vi "pointage.vi"() -> ()   [LabVIEW 2024]
uses:
  <vilib>/drjdpowell/SQLite Library/SQL Connection/Open (string).vi
  <vilib>/drjdpowell/SQLite Library/SQL Connection/Execute SQL (No results).vi
  <vilib>/drjdpowell/SQLite Library/SQL Connection/Execute SQL.vi
  <vilib>/drjdpowell/SQLite Library/SQL Connection/Connection.lvclass
  <vilib>/drjdpowell/SQLite Library/SQLite.lvlib
panel:
  out "Données pointage":string[][](table)
  out "Heure":string
  out "Identifiant":dbl
  in  "Heure":timestamp
  in  "Identifiant":dbl
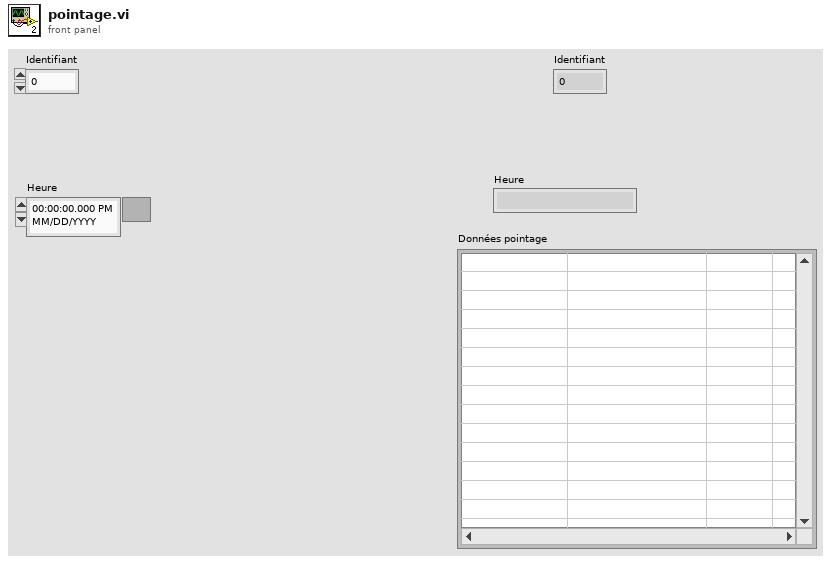
[diagram p1: front panel]
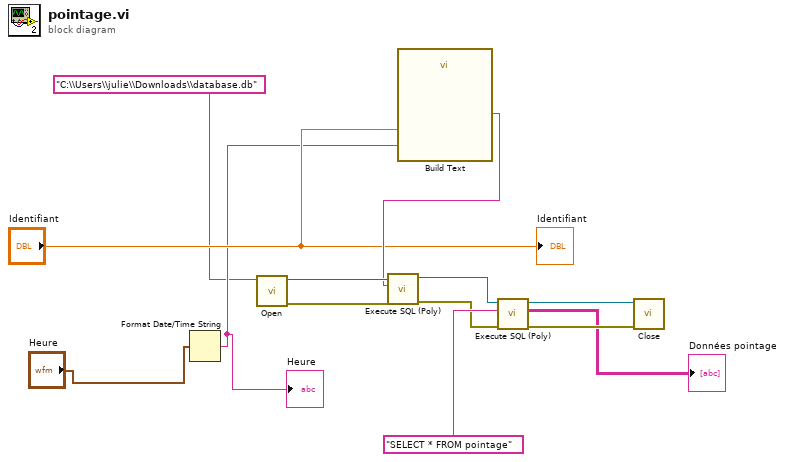
[diagram p0: block diagram]
diagram:
  n1 = Format Date/Time String(seconds (now)="Heure") -> (date/time string=w8:string)  [unwired: 2 in]
  "Heure" <- w8
  n2 = call-poly <vilib>:"Open.vi"("db file"="C:\\Users\\julie\\Downloads\\database.db") -> ("error out"=w11:errorcluster, "SQLite Connection"=w12:refnum<class "Connection.lvclass">)  [unwired: 9 in]
  n3 = call "Build Text"("id"="Identifiant", "heure"=w8) -> ("Result"=w10:string)  [unwired: 12 in, 1 out]
  n4 = call-poly <vilib>:"Execute SQL (Poly).vi"("error in (no error)"=w11, "SQL"=w10, "SQLite Connection in"=w12) -> ("error out"=w1:errorcluster, "SQLite Connection"=w2:refnum<class "Connection.lvclass">)  [unwired: 7 in]
  n5 = call-poly <vilib>:"Execute SQL (Poly).vi"("error in (no error)"=w1, "SQL"="SELECT * FROM pointage", "SQLite Connection in"=w2) -> ("error out"=w5:errorcluster, "Result Set"=→"Données pointage":string[][], "SQLite Connection"=w6:refnum<class "Connection.lvclass">)  [unwired: 5 in, 1 out]
  n6 = call-dynamic "Close.vi"("error in (no error)"=w5, "SQLite Connection in"=w6) -> ()  [unwired: 9 in, 1 out]
  "Identifiant" <- "Identifiant"
